vi "read_params.vi"(8 "error in (no error)":errorcluster, 11 "VotingRegressor in":refnum<class "VotingRegressor.lvclass">) -> (0 "error out":errorcluster, 2 "params":T1={"estimators"=[], "weights"={"weights_type"="None", "weights_list"=[]}, "n_jobs"=1.0, "verbose"=FALSE}, 3 "VotingRegressor out":refnum<class "VotingRegressor.lvclass">)   [LabVIEW 2020, in "VotingRegressor.lvclass"]
uses:
  VotingRegressor.lvclass
  Controls/voting_regressor_params.ctl
  VotingRegressor.lvclass/VotingRegressor.ctl
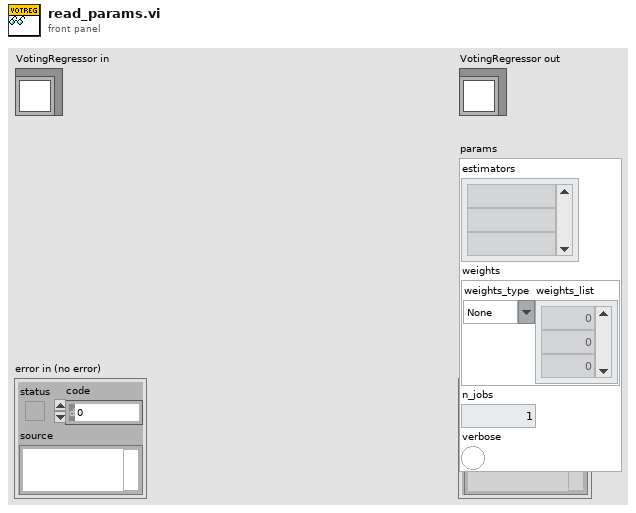
[diagram p1: front panel]
types:
  T1 = typedef "voting_regressor_params.ctl" = cluster{"estimators":string[], "weights":cluster{"weights_type":string, "weights_list":dbl[]}, "n_jobs":dbl, "verbose":bool}
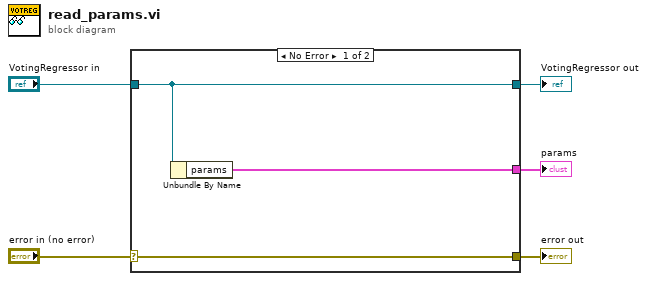
[diagram p0: block diagram]
diagram:
  n1 = case shown="No Error" "error in (no error)" {
    selector: "error in (no error)" -> [w8 w9]
    tunnel: [w8 w9] -> w4
    tunnel: [w7 w10] -> w2
    tunnel: "VotingRegressor in" -> [w7 w10]
    tunnel: [w6 _] -> w1
    frame No Error {
      n2 = Unbundle By Name(w7) -> ("params"=w6:T1)
    }
    frame Error {
    }
  }
  "error out" <- w4
  "VotingRegressor out" <- w2
  "params" <- w1
